vi "Camera Status Callback.vi"(4 "Camera_Prime95B in":refnum<class "Camera_Prime95B.lvclass">, 5 "Event Data":cluster{"sender":refnum<k24>, "e":refnum<k24>}, 6 "Control Ref":refnum<k24>, 7 "Event Common Data":T1) -> ()   [LabVIEW 2020, in "Camera_Prime95B.lvlib" / "Camera_Prime95B.lvclass"]
uses:
  Camera_Prime95B.lvclass
  C:/Program Files/National Instruments/LabVIEW 2020/vi.lib/ActorFramework/Actor/Actor.lvclass
  D:/Daguan/Development/MMicroscopyAF/Model/Real Hardware/Camera_Prime95B/Camera_Prime95B/Dependencies/PVCamNET.dll
  Dependencies/PVCamNET.dll
  <vilib>/ActorFramework/Actor/Actor.lvclass/Actor.ctl
  <vilib>/ActorFramework/Message Enqueuer/Message Enqueuer.lvclass/Message Enqueuer.ctl
  <vilib>/ActorFramework/Message Enqueuer/Init from Existing Queue.vi
  <vilib>/ActorFramework/Message Enqueuer/Enqueue.vi
  Camera_Prime95B Messages/On Acquisition Stop Msg/On Acquisition Stop Msg.lvclass
  C:/Program Files/National Instruments/LabVIEW 2020/vi.lib/ActorFramework/Message/Message.lvclass
  <vilib>/ActorFramework/Message Priority Queue/Priority Enqueue.vi
  <vilib>/ActorFramework/Message Enqueuer/Message Enqueuer.lvclass
  <vilib>/ActorFramework/Actor/Actor.lvclass
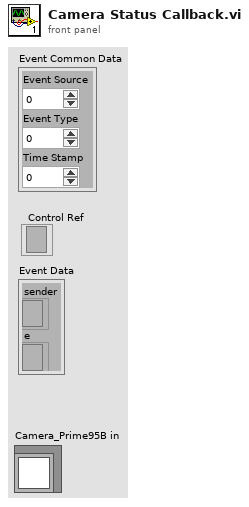
[diagram p1: front panel]
types:
  T1 = cluster{"Event Source":i32, "Event Type":u32, "Time Stamp":u32}
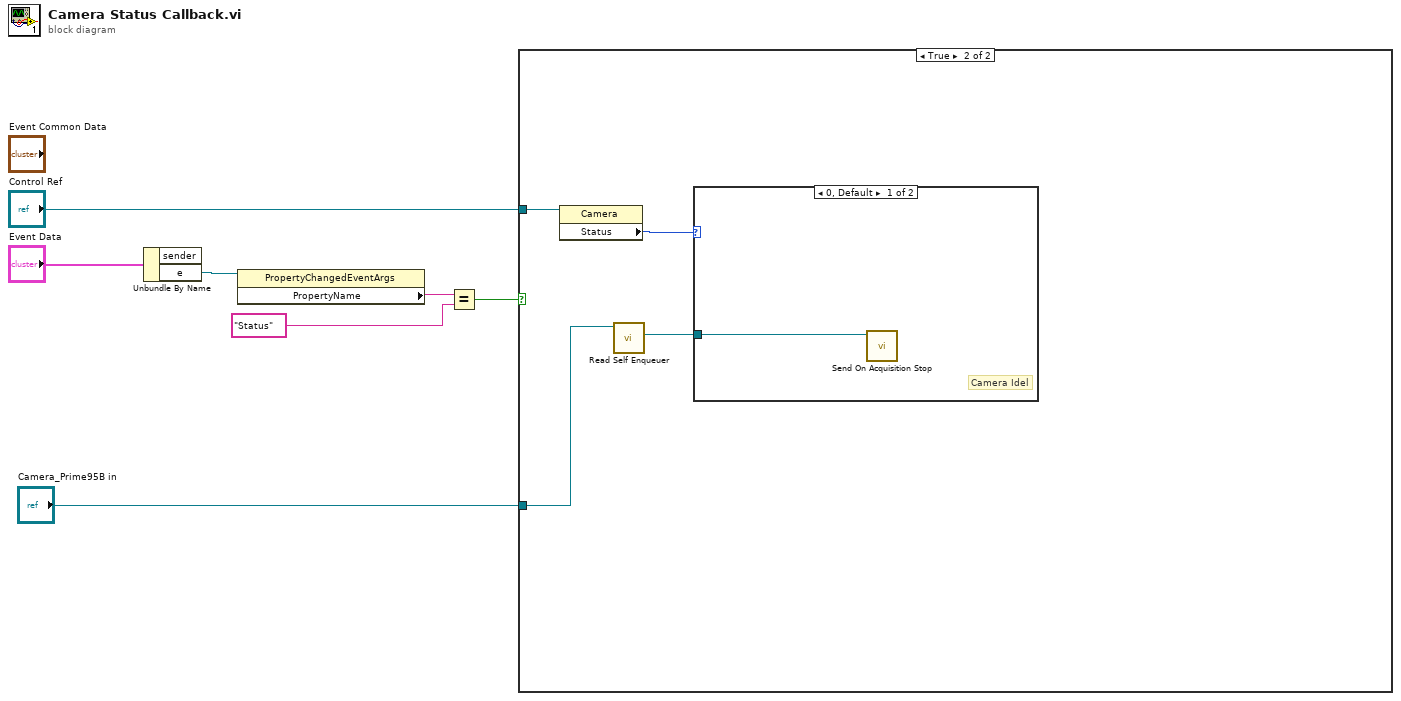
[diagram p0: block diagram]
diagram:
  n1 = Unbundle By Name("Event Data") -> ("e"=w6:refnum<k24>)  [unwired: 1 out]
  n2 = property class="PropertyChangedEventArgs"(reference=w6) -> ("PropertyName"=w5:string)  [unwired: 1 in, 2 out]
  n3 = Equal?(x=w5, y="Status") -> (x = y?=w3:bool)
  n4 = case shown="True" w3 {
    tunnel: "Control Ref" -> [_ w11]
    tunnel: "Camera_Prime95B in" -> [_ w9]
    frame False {
    }
    frame True {
      n5 = property class="Camera"(reference=w11) -> ("Status"=w10:i32)  [unwired: 1 in, 2 out]
      n6 = call <vilib>:"Read Self Enqueuer.vi"("Actor"=w9) -> ("Self Enqueuer"=w8:refnum<class "Message Enqueuer.lvclass">)  [unwired: 10 in]
      n7 = case shown="0, Default" w10 {
        tunnel: w8 -> [w12 _]
        frame 0, Default {
          # "Camera Idel"
          n8 = call "Send On Acquisition Stop.vi"("Message Enqueuer"=w12) -> ()  [unwired: 9 in, 2 out]
        }
        frame 1 {
        }
      }
    }
  }
